vi "Add Triggers and Buffer IDs to Acyclic Frames.vi"(8 "error in":errorcluster, 10 "acyclic frame names":string[](array[string]), 11 "acyclic frames section":T1=18446744073709551615 format="%.0x") -> (0 "error out":errorcluster, 3 "acyclic frames section out":T1=18446744073709551615 format="%.0x")   [LabVIEW 2020, in "AIM MIL-STD-1553 Scripting.lvlib"]
doc: "Adds an Acyclic Frame Trigger to each of the Acyclic Frames in the <b>acyclic frames section</b> that are specified in <b>acyclic frame names</b>."
uses:
  AIM MIL-STD-1553 Scripting.lvlib
  <vilib>/NI VeriStand/Custom Device API/Custom Device Item Ref.ctl
  Constants.vi
  <vilib>/NI VeriStand/Custom Device API/Custom Device API.lvlib
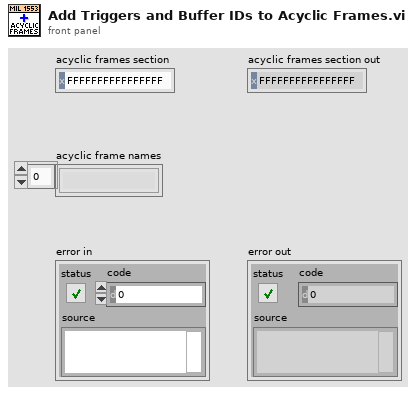
[diagram p1: front panel]
types:
  T1 = typedef "Custom Device API.lvlib/Custom Device Item Ref.ctl" = u64
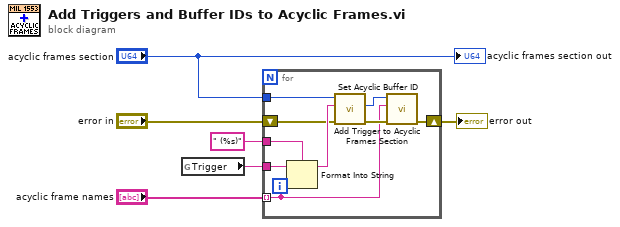
[diagram p0: block diagram]
diagram:
  n1 = global read "Constants.vi" "Trigger"() -> (w6:string)
  n2 = for {
    tunnel: w6 -> [w15]
    tunnel: " (%s)" ("format string") -> [w14]
    shift-right: [w9] -> w4
    shift-left: "error in" -> [w12]
    tunnel: "acyclic frame names" -> [w8] mode=indexing
    tunnel: "acyclic frames section" -> [w11]
    n3 = Format Into String(format string=w14, initial string=w15, w8) -> (resulting string=w13:string)  [unwired: 1 in, 1 out]
    n4 = call "Add Trigger to Acyclic Frames Section.vi"("error in"=w12, "trigger name"=w13, "acyclic frames section"=w11) -> ("error out"=w10:errorcluster, "acyclic frame trigger"=w7:T1)  [unwired: 6 in, 1 out]
    n5 = call "Set Acyclic Buffer ID.vi"("error in"=w10, "acyclic buffer id"=w8, "acyclic frame trigger"=w7) -> ("error out"=w9:errorcluster)  [unwired: 7 in, 1 out]
  }
  "error out" <- w4
  "acyclic frames section out" <- "acyclic frames section"
